vi "LCDCopy.vi"(0 "Device In":u64, 1 "srcX1":i32, 2 "srcY1":i32, 3 "srcX2":i32, 4 "srcY2":i32, 5 "error in (no error)":errorcluster, 6 "srcFramebuffer":i32, 7 "inverted":i32, 8 "dstFramebuffer":i32, 10 "dstX":i32, 12 "dstY":i32) -> (14 "Device Out":u64, 19 "error out":errorcluster)   [LabVIEW 2012, in "Phidget LCD.lvlib"]
doc: "${Copy:Header}"
uses:
  <instrlib>/Phidgets/Phidget LCD/Phidget LCD.lvlib
  <instrlib>/Phidgets/Phidget Common/Phidget Common.lvlib
  phidget22.dll
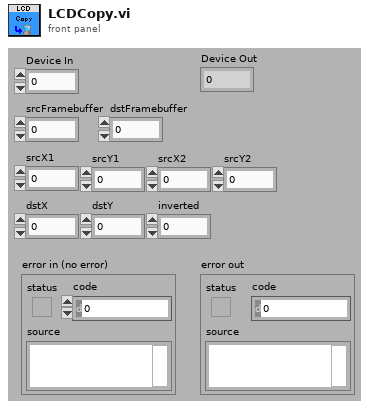
[diagram p1: front panel]
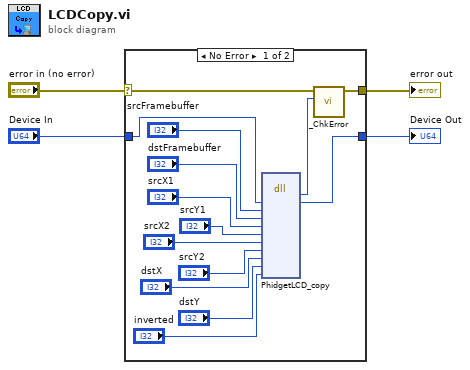
[diagram p0: block diagram]
diagram:
  n1 = case shown="No Error" "error in (no error)" {
    selector: "error in (no error)" -> [w18 w20]
    tunnel: [w17 w20] -> w3
    tunnel: "Device In" -> [w16 w19]
    tunnel: [w15 w19] -> w1
    frame No Error {
      n2 = dll-call lib="phidget22.*" fn="PhidgetLCD_copy"("phid"=w16, "srcFramebuffer"="srcFramebuffer", "dstFramebuffer"="dstFramebuffer", "srcX1"="srcX1", "srcY1"="srcY1", "srcX2"="srcX2", "srcY2"="srcY2", "dstX"="dstX", "dstY"="dstY", "inverted"="inverted") -> ("return type"=w14:i32, "phid"=w15:u64)  [unwired: 12 in, 2 out]
      n3 = call <instrlib>:"_ChkError.vi"("Return Code"=w14, "error in (no error)"=w18) -> ("error out"=w17:errorcluster)  [unwired: 9 in]
    }
    frame Error {
    }
  }
  "error out" <- w3
  "Device Out" <- w1
